vi "Modbus Real Time Clock.vi"(0 "Month":i16, 1 "Year":i16, 5 "Day":i16, 7 "Hour":i16, 9 "Minute":i16, 11 "Second":i16) -> (4 "Real-Time Clock":T1, 6 "Absolute Time":dbl format="%<%H:%M:%S%3u>t")   [LabVIEW 2020, in "Modbus.lvlib"]
uses:
  Modbus.lvlib
  <vilib>/Utility/miscctls.llb/LVDateTimeRec.ctl
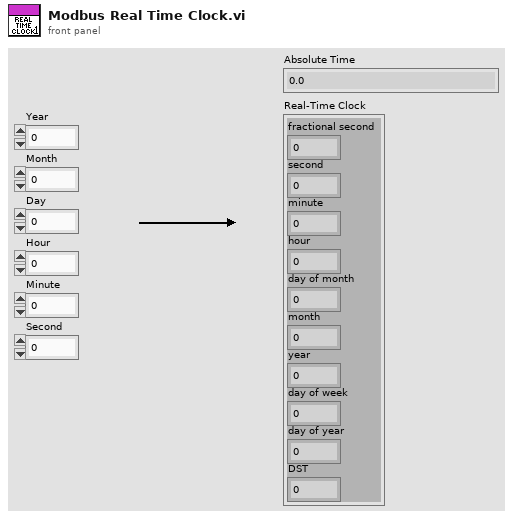
[diagram p1: front panel]
types:
  T1 = typedef "LVDateTimeRec.ctl" = cluster{"fractional second":dbl, "second":i32, "minute":i32, "hour":i32, "day of month":i32, "month":i32, "year":i32, "day of week":i32, "day of year":i32, "DST":i32}
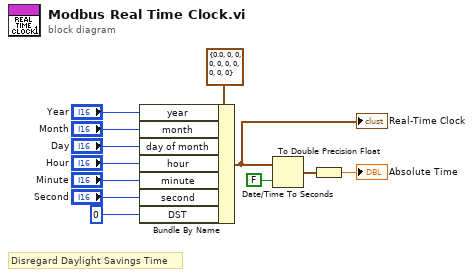
[diagram p0: block diagram]
diagram:
  # "Disregard Daylight Savings Time"
  n1 = Bundle By Name(cluster=T1 {"fractional second"=0.0, "second"=0, "minute"=0, "hour"=0, "day of month"=0, "month"=0, "year"=0, "day of week"=0, "day of year"=0, "DST"=0} ("date time rec"), "year"="Year", "month"="Month", "day of month"="Day", "hour"="Hour", "minute"="Minute", "second"="Second", "DST"=0) -> (w11:T1)
  "Real-Time Clock" <- w11
  n2 = Date/Time To Seconds(1:FALSE ("is UTC (F)"), 2:w11) -> (0:w10:timestamp)
  n3 = To Double Precision Float(number=w10) -> (double precision float=→"Absolute Time":dbl)
